vi "電梯2.vi"() -> ()   [LabVIEW 2021]
panel:
  out "時間":string
  out "日期":string
  out "訊息":string
  out "現在樓層":i32
  in  "四樓":bool
  in  "三樓":bool
  in  "二樓":bool
  in  "一樓":bool
  in  "緊急停止":bool
  in  "延長開關":bool
  out "傳感器":bool
  out "樓層位置":i32[](array[numeric])
  in  "程式結束":bool
  out "呼叫樓層":i32
  out "顯示樓層":i32(knob) scale=1.0..4.0
  out "緊急停止燈":bool
  out "顯示燈 4":bool
  out "顯示燈 3":bool
  out "顯示燈 2":bool
  out "顯示燈":bool
  out "電梯門 4":u16(ring)
  out "電梯門 3":u16(ring)
  out "電梯門 2":u16(ring)
  out "電梯門":u16(ring)
  out "電梯位置":i32(slide) scale=0.0..4.0
  in  "呼叫鈕4":bool
  in  "呼叫鈕3":bool
  in  "呼叫鈕2":bool
  in  "呼叫鈕":bool
  # "4"
  # "3"
  # "2"
  # "1"
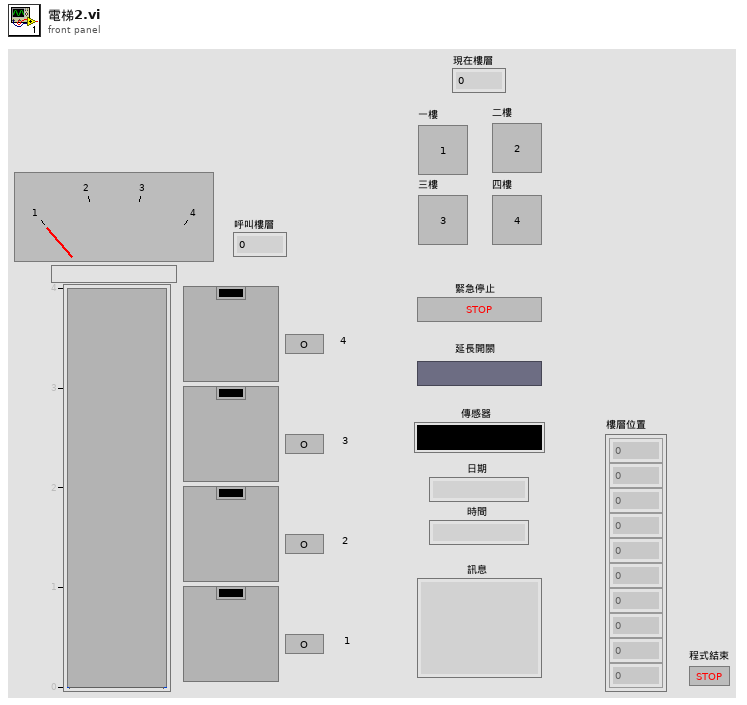
[diagram p1: front panel]
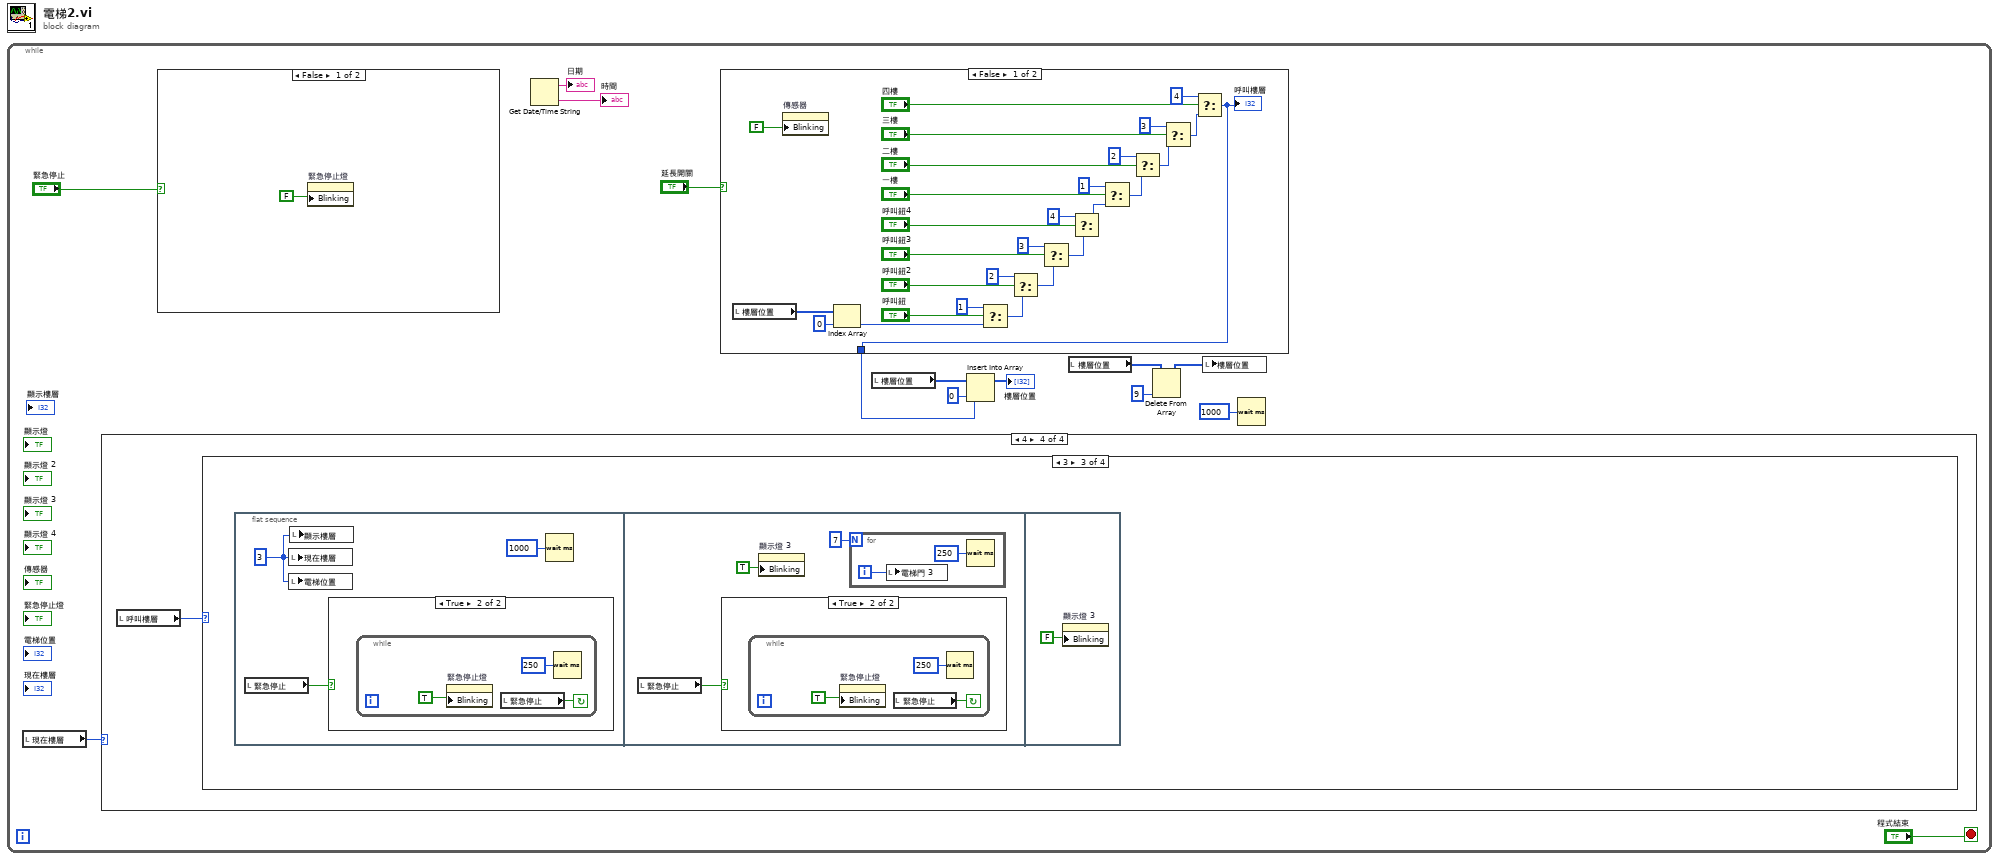
[diagram p0: block diagram]
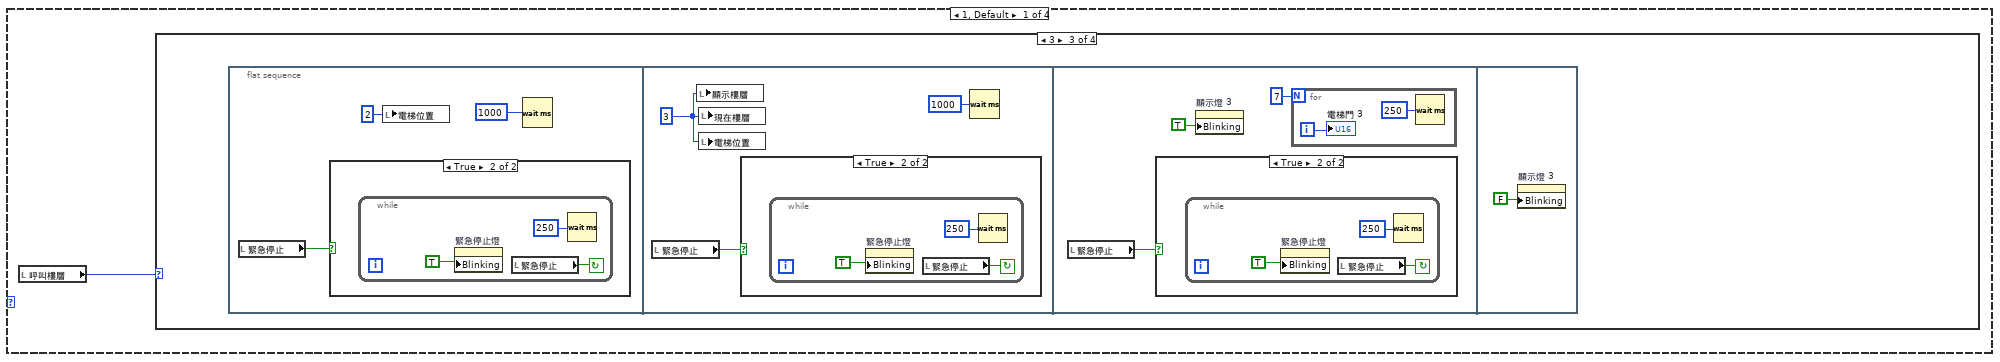
[diagram p2: hidden frame]
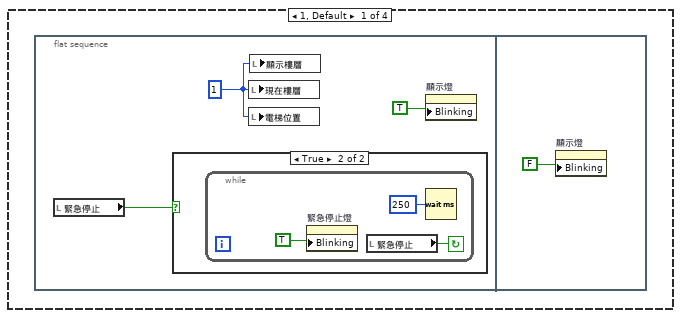
[diagram p3: hidden frame]
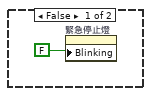
[diagram p4: hidden frame]
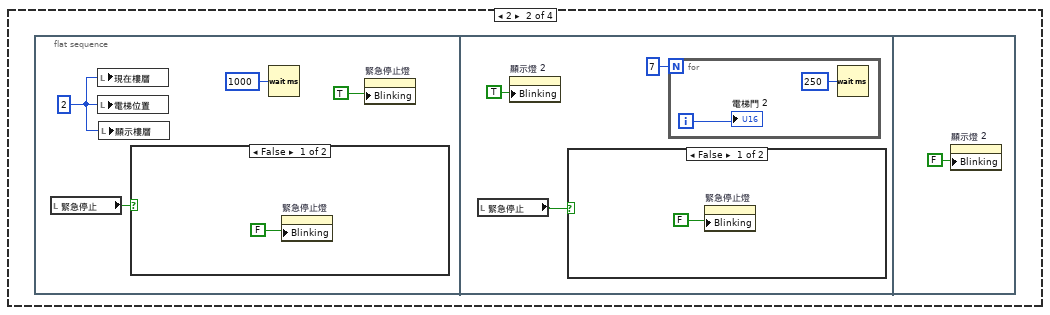
[diagram p5: hidden frame]
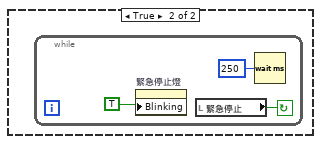
[diagram p6: hidden frame]
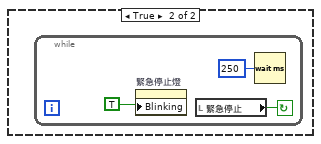
[diagram p7: hidden frame]
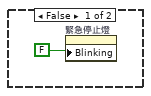
[diagram p8: hidden frame]
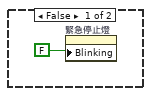
[diagram p9: hidden frame]
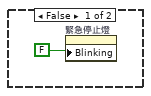
[diagram p10: hidden frame]
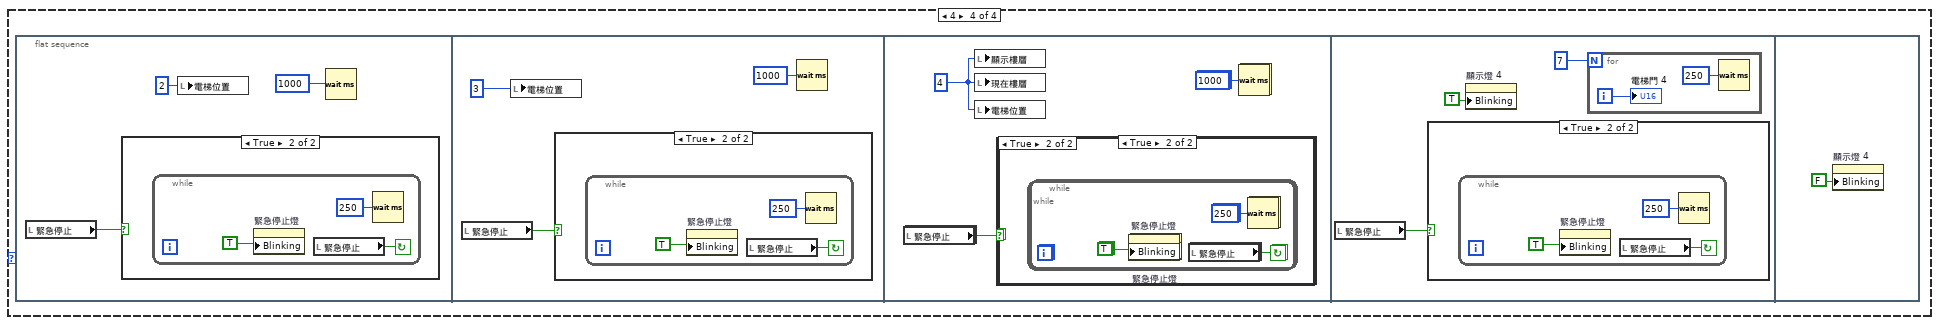
[diagram p11: hidden frame]
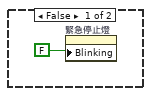
[diagram p12: hidden frame]
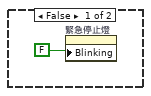
[diagram p13: hidden frame]
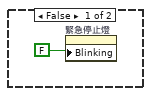
[diagram p14: hidden frame]
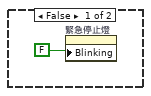
[diagram p15: hidden frame]
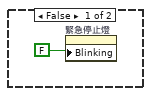
[diagram p16: hidden frame]
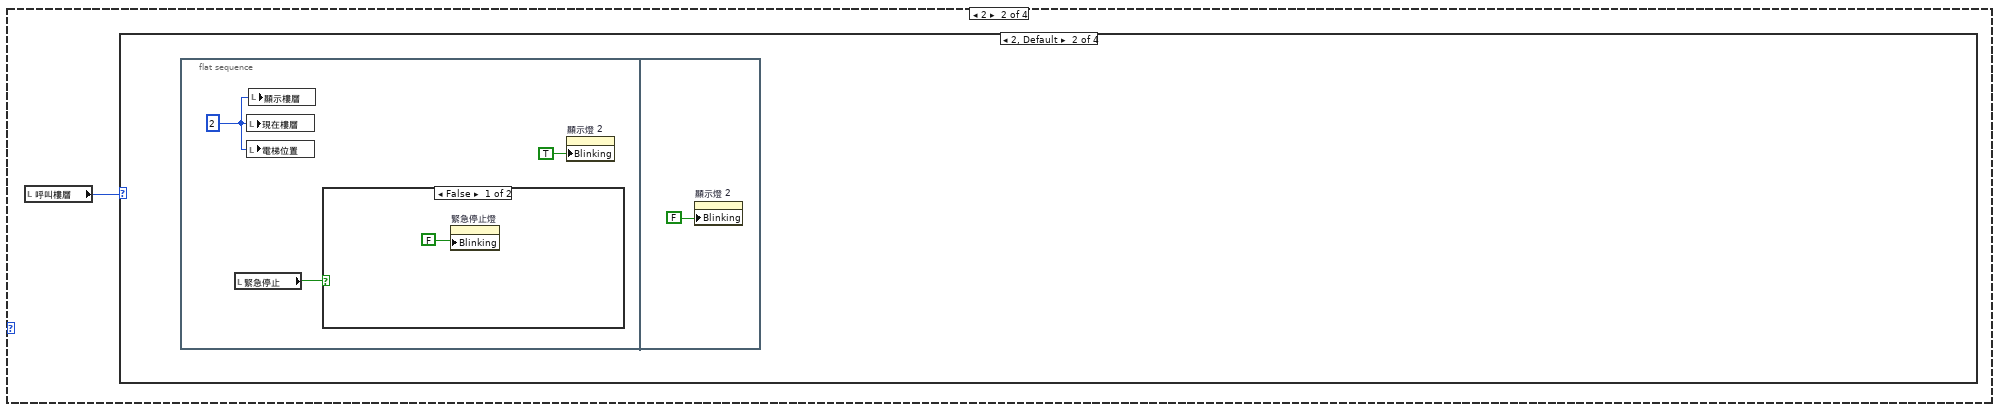
[diagram p17: hidden frame]
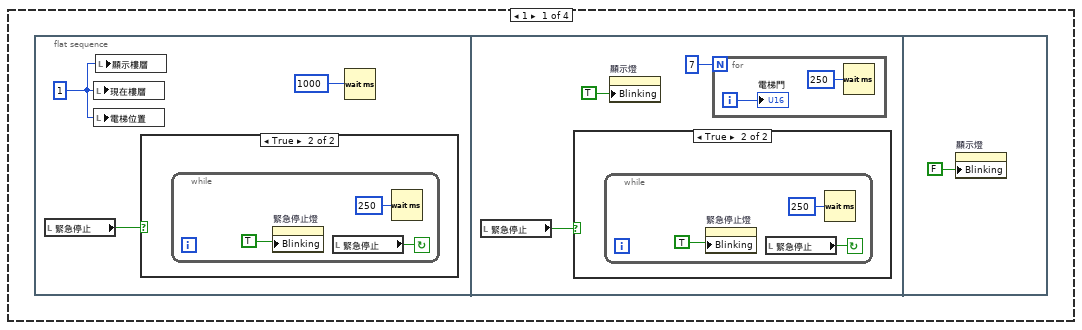
[diagram p18: hidden frame]
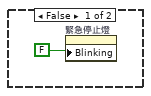
[diagram p19: hidden frame]
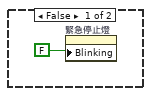
[diagram p20: hidden frame]
diagram:
  n1 = while {
    stop <- "程式結束" stop-if-true
    n2 = local read "現在樓層"() -> (w4:i32)
    n3 = case shown="4" w4 {
      frame 1, Default {
        n4 = local read "呼叫樓層"() -> (w15:i32)
        n5 = case shown="3" w15 {
          frame 1, Default {
            n6 = flat-sequence {
              frame #0 {
                w16 = 1
                n7 = local read "緊急停止"() -> (w18:bool)
                n8 = case shown="True" w18 {
                  frame False {
                    n9 = property on="緊急停止燈" class="Bool (strict)"("Blinking"=FALSE) -> ()  [unwired: 2 in, 2 out]
                  }
                  frame True {
                    n10 = while {
                      stop <- w22 continue-if-true
                      n11 = property on="緊急停止燈" class="Bool (strict)"("Blinking"=TRUE) -> ()  [unwired: 2 in, 2 out]
                      n12 = local read "緊急停止"() -> (w22:bool)
                      n13 = Wait (ms)(milliseconds to wait=u32 250) -> ()  [unwired: 1 out]
                    }
                  }
                }
                n14 = local write "現在樓層"(w16) -> ()
                n15 = local write "電梯位置"(w16) -> ()
                n16 = local write "顯示樓層"(w16) -> ()
                n17 = property on="顯示燈" class="Bool (strict)"("Blinking"=TRUE) -> ()  [unwired: 2 in, 2 out]
              }
              frame #1 {
                n18 = property on="顯示燈" class="Bool (strict)"("Blinking"=FALSE) -> ()  [unwired: 2 in, 2 out]
              }
            }
          }
          frame 2 {
            n19 = flat-sequence {
              frame #0 {
                w24 = 2
                n20 = local read "緊急停止"() -> (w27:bool)
                n21 = local write "現在樓層"(w24) -> ()
                n22 = local write "電梯位置"(w24) -> ()
                n23 = local write "顯示樓層"(w24) -> ()
                n24 = case shown="False" w27 {
                  frame False {
                    n25 = property on="緊急停止燈" class="Bool (strict)"("Blinking"=FALSE) -> ()  [unwired: 2 in, 2 out]
                  }
                  frame True {
                    n26 = while {
                      stop <- w31 continue-if-true
                      n27 = property on="緊急停止燈" class="Bool (strict)"("Blinking"=TRUE) -> ()  [unwired: 2 in, 2 out]
                      n28 = local read "緊急停止"() -> (w31:bool)
                      n29 = Wait (ms)(milliseconds to wait=u32 250) -> ()  [unwired: 1 out]
                    }
                  }
                }
                n30 = Wait (ms)(milliseconds to wait=u32 1000) -> ()  [unwired: 1 out]
                n31 = property on="緊急停止燈" class="Bool (strict)"("Blinking"=TRUE) -> ()  [unwired: 2 in, 2 out]
              }
              frame #1 {
                n32 = local read "緊急停止"() -> (w34:bool)
                n33 = property on="顯示燈 2" class="Bool (strict)"("Blinking"=TRUE) -> ()  [unwired: 2 in, 2 out]
                n34 = case shown="False" w34 {
                  frame False {
                    n35 = property on="緊急停止燈" class="Bool (strict)"("Blinking"=FALSE) -> ()  [unwired: 2 in, 2 out]
                  }
                  frame True {
                    n36 = while {
                      stop <- w40 continue-if-true
                      n37 = property on="緊急停止燈" class="Bool (strict)"("Blinking"=TRUE) -> ()  [unwired: 2 in, 2 out]
                      n38 = local read "緊急停止"() -> (w40:bool)
                      n39 = Wait (ms)(milliseconds to wait=u32 250) -> ()  [unwired: 1 out]
                    }
                  }
                }
                n40 = for {
                  N: 7 -> [_]
                  i -> [w35]
                  n41 = Wait (ms)(milliseconds to wait=u32 250) -> ()  [unwired: 1 out]
                  "電梯門 2" <- w35
                }
              }
              frame #2 {
                n42 = property on="顯示燈 2" class="Bool (strict)"("Blinking"=FALSE) -> ()  [unwired: 2 in, 2 out]
              }
            }
          }
          frame 3 {
            n43 = flat-sequence {
              frame #0 {
                n44 = local read "緊急停止"() -> (w44:bool)
                n45 = case shown="True" w44 {
                  frame False {
                    n46 = property on="緊急停止燈" class="Bool (strict)"("Blinking"=FALSE) -> ()  [unwired: 2 in, 2 out]
                  }
                  frame True {
                    n47 = while {
                      stop <- w48 continue-if-true
                      n48 = property on="緊急停止燈" class="Bool (strict)"("Blinking"=TRUE) -> ()  [unwired: 2 in, 2 out]
                      n49 = local read "緊急停止"() -> (w48:bool)
                      n50 = Wait (ms)(milliseconds to wait=u32 250) -> ()  [unwired: 1 out]
                    }
                  }
                }
                n51 = local write "電梯位置"(2 ("電梯位置")) -> ()
                n52 = Wait (ms)(milliseconds to wait=u32 1000) -> ()  [unwired: 1 out]
              }
              frame #1 {
                w49 = 3
                n53 = local read "緊急停止"() -> (w51:bool)
                n54 = local write "顯示樓層"(w49) -> ()
                n55 = local write "現在樓層"(w49) -> ()
                n56 = local write "電梯位置"(w49) -> ()
                n57 = case shown="True" w51 {
                  frame False {
                    n58 = property on="緊急停止燈" class="Bool (strict)"("Blinking"=FALSE) -> ()  [unwired: 2 in, 2 out]
                  }
                  frame True {
                    n59 = while {
                      stop <- w55 continue-if-true
                      n60 = property on="緊急停止燈" class="Bool (strict)"("Blinking"=TRUE) -> ()  [unwired: 2 in, 2 out]
                      n61 = local read "緊急停止"() -> (w55:bool)
                      n62 = Wait (ms)(milliseconds to wait=u32 250) -> ()  [unwired: 1 out]
                    }
                  }
                }
                n63 = Wait (ms)(milliseconds to wait=u32 1000) -> ()  [unwired: 1 out]
              }
              frame #2 {
                n64 = local read "緊急停止"() -> (w58:bool)
                n65 = case shown="True" w58 {
                  frame False {
                    n66 = property on="緊急停止燈" class="Bool (strict)"("Blinking"=FALSE) -> ()  [unwired: 2 in, 2 out]
                  }
                  frame True {
                    n67 = while {
                      stop <- w64 continue-if-true
                      n68 = property on="緊急停止燈" class="Bool (strict)"("Blinking"=TRUE) -> ()  [unwired: 2 in, 2 out]
                      n69 = local read "緊急停止"() -> (w64:bool)
                      n70 = Wait (ms)(milliseconds to wait=u32 250) -> ()  [unwired: 1 out]
                    }
                  }
                }
                n71 = property on="顯示燈 3" class="Bool (strict)"("Blinking"=TRUE) -> ()  [unwired: 2 in, 2 out]
                n72 = for {
                  N: 7 -> [_]
                  i -> [w60]
                  n73 = Wait (ms)(milliseconds to wait=u32 250) -> ()  [unwired: 1 out]
                  "電梯門 3" <- w60
                }
              }
              frame #3 {
                n74 = property on="顯示燈 3" class="Bool (strict)"("Blinking"=FALSE) -> ()  [unwired: 2 in, 2 out]
              }
            }
          }
          frame 4 {
            n75 = flat-sequence {
              frame #0 {
                n76 = local read "緊急停止"() -> (w68:bool)
                n77 = case shown="True" w68 {
                  frame False {
                    n78 = property on="緊急停止燈" class="Bool (strict)"("Blinking"=FALSE) -> ()  [unwired: 2 in, 2 out]
                  }
                  frame True {
                    n79 = while {
                      stop <- w72 continue-if-true
                      n80 = property on="緊急停止燈" class="Bool (strict)"("Blinking"=TRUE) -> ()  [unwired: 2 in, 2 out]
                      n81 = local read "緊急停止"() -> (w72:bool)
                      n82 = Wait (ms)(milliseconds to wait=u32 250) -> ()  [unwired: 1 out]
                    }
                  }
                }
                n83 = local write "電梯位置"(2 ("電梯位置")) -> ()
                n84 = Wait (ms)(milliseconds to wait=u32 1000) -> ()  [unwired: 1 out]
              }
              frame #1 {
                n85 = local read "緊急停止"() -> (w75:bool)
                n86 = local write "電梯位置"(3) -> ()
                n87 = case shown="True" w75 {
                  frame False {
                    n88 = property on="緊急停止燈" class="Bool (strict)"("Blinking"=FALSE) -> ()  [unwired: 2 in, 2 out]
                  }
                  frame True {
                    n89 = while {
                      stop <- w79 continue-if-true
                      n90 = property on="緊急停止燈" class="Bool (strict)"("Blinking"=TRUE) -> ()  [unwired: 2 in, 2 out]
                      n91 = local read "緊急停止"() -> (w79:bool)
                      n92 = Wait (ms)(milliseconds to wait=u32 250) -> ()  [unwired: 1 out]
                    }
                  }
                }
                n93 = Wait (ms)(milliseconds to wait=u32 1000) -> ()  [unwired: 1 out]
              }
              frame #2 {
                w80 = 4
                n94 = local read "緊急停止"() -> (w83:bool)
                n95 = local read "緊急停止"() -> (w82:bool)
                n96 = local write "顯示樓層"(w80) -> ()
                n97 = local write "現在樓層"(w80) -> ()
                n98 = local write "電梯位置"(w80) -> ()
                n99 = case shown="True" w83 {
                  frame False {
                    n100 = property on="緊急停止燈" class="Bool (strict)"("Blinking"=FALSE) -> ()  [unwired: 2 in, 2 out]
                  }
                  frame True {
                    n101 = while {
                      stop <- w92 continue-if-true
                      n102 = property on="緊急停止燈" class="Bool (strict)"("Blinking"=TRUE) -> ()  [unwired: 2 in, 2 out]
                      n103 = local read "緊急停止"() -> (w92:bool)
                      n104 = Wait (ms)(milliseconds to wait=u32 250) -> ()  [unwired: 1 out]
                    }
                  }
                }
                n105 = case shown="True" w82 {
                  frame False {
                    n106 = property on="緊急停止燈" class="Bool (strict)"("Blinking"=FALSE) -> ()  [unwired: 2 in, 2 out]
                  }
                  frame True {
                    n107 = while {
                      stop <- w88 continue-if-true
                      n108 = property on="緊急停止燈" class="Bool (strict)"("Blinking"=TRUE) -> ()  [unwired: 2 in, 2 out]
                      n109 = local read "緊急停止"() -> (w88:bool)
                      n110 = Wait (ms)(milliseconds to wait=u32 250) -> ()  [unwired: 1 out]
                    }
                  }
                }
                n111 = Wait (ms)(milliseconds to wait=u32 1000) -> ()  [unwired: 1 out]
                n112 = Wait (ms)(milliseconds to wait=u32 1000) -> ()  [unwired: 1 out]
              }
              frame #3 {
                n113 = local read "緊急停止"() -> (w95:bool)
                n114 = case shown="True" w95 {
                  frame False {
                    n115 = property on="緊急停止燈" class="Bool (strict)"("Blinking"=FALSE) -> ()  [unwired: 2 in, 2 out]
                  }
                  frame True {
                    n116 = while {
                      stop <- w101 continue-if-true
                      n117 = property on="緊急停止燈" class="Bool (strict)"("Blinking"=TRUE) -> ()  [unwired: 2 in, 2 out]
                      n118 = local read "緊急停止"() -> (w101:bool)
                      n119 = Wait (ms)(milliseconds to wait=u32 250) -> ()  [unwired: 1 out]
                    }
                  }
                }
                n120 = property on="顯示燈 4" class="Bool (strict)"("Blinking"=TRUE) -> ()  [unwired: 2 in, 2 out]
                n121 = for {
                  N: 7 -> [_]
                  i -> [w96]
                  n122 = Wait (ms)(milliseconds to wait=u32 250) -> ()  [unwired: 1 out]
                  "電梯門 4" <- w96
                }
              }
              frame #4 {
                n123 = property on="顯示燈 4" class="Bool (strict)"("Blinking"=FALSE) -> ()  [unwired: 2 in, 2 out]
              }
            }
          }
        }
      }
      frame 2 {
        n124 = local read "呼叫樓層"() -> (w103:i32)
        n125 = case shown="2, Default" w103 {
          frame 1 {
            n126 = flat-sequence {
              frame #0 {
                w104 = 1
                n127 = local read "緊急停止"() -> (w106:bool)
                n128 = local write "現在樓層"(w104) -> ()
                n129 = local write "電梯位置"(w104) -> ()
                n130 = local write "顯示樓層"(w104) -> ()
                n131 = case shown="True" w106 {
                  frame False {
                    n132 = property on="緊急停止燈" class="Bool (strict)"("Blinking"=FALSE) -> ()  [unwired: 2 in, 2 out]
                  }
                  frame True {
                    n133 = while {
                      stop <- w110 continue-if-true
                      n134 = property on="緊急停止燈" class="Bool (strict)"("Blinking"=TRUE) -> ()  [unwired: 2 in, 2 out]
                      n135 = local read "緊急停止"() -> (w110:bool)
                      n136 = Wait (ms)(milliseconds to wait=u32 250) -> ()  [unwired: 1 out]
                    }
                  }
                }
                n137 = Wait (ms)(milliseconds to wait=u32 1000) -> ()  [unwired: 1 out]
              }
              frame #1 {
                n138 = local read "緊急停止"() -> (w113:bool)
                n139 = case shown="True" w113 {
                  frame False {
                    n140 = property on="緊急停止燈" class="Bool (strict)"("Blinking"=FALSE) -> ()  [unwired: 2 in, 2 out]
                  }
                  frame True {
                    n141 = while {
                      stop <- w119 continue-if-true
                      n142 = property on="緊急停止燈" class="Bool (strict)"("Blinking"=TRUE) -> ()  [unwired: 2 in, 2 out]
                      n143 = local read "緊急停止"() -> (w119:bool)
                      n144 = Wait (ms)(milliseconds to wait=u32 250) -> ()  [unwired: 1 out]
                    }
                  }
                }
                n145 = property on="顯示燈" class="Bool (strict)"("Blinking"=TRUE) -> ()  [unwired: 2 in, 2 out]
                n146 = for {
                  N: 7 -> [_]
                  i -> [w114]
                  n147 = Wait (ms)(milliseconds to wait=u32 250) -> ()  [unwired: 1 out]
                  "電梯門" <- w114
                }
              }
              frame #2 {
                n148 = property on="顯示燈" class="Bool (strict)"("Blinking"=FALSE) -> ()  [unwired: 2 in, 2 out]
              }
            }
          }
          frame 2, Default {
            n149 = flat-sequence {
              frame #0 {
                w121 = 2
                n150 = local read "緊急停止"() -> (w123:bool)
                n151 = local write "現在樓層"(w121) -> ()
                n152 = local write "電梯位置"(w121) -> ()
                n153 = local write "顯示樓層"(w121) -> ()
                n154 = case shown="False" w123 {
                  frame False {
                    n155 = property on="緊急停止燈" class="Bool (strict)"("Blinking"=FALSE) -> ()  [unwired: 2 in, 2 out]
                  }
                  frame True {
                    n156 = while {
                      stop <- w127 continue-if-true
                      n157 = property on="緊急停止燈" class="Bool (strict)"("Blinking"=TRUE) -> ()  [unwired: 2 in, 2 out]
                      n158 = local read "緊急停止"() -> (w127:bool)
                      n159 = Wait (ms)(milliseconds to wait=u32 250) -> ()  [unwired: 1 out]
                    }
                  }
                }
                n160 = property on="顯示燈 2" class="Bool (strict)"("Blinking"=TRUE) -> ()  [unwired: 2 in, 2 out]
              }
              frame #1 {
                n161 = property on="顯示燈 2" class="Bool (strict)"("Blinking"=FALSE) -> ()  [unwired: 2 in, 2 out]
              }
            }
          }
          frame 3 {
            n162 = flat-sequence {
              frame #0 {
                w129 = 3
                n163 = local read "緊急停止"() -> (w130:bool)
                n164 = local write "現在樓層"(w129) -> ()
                n165 = local write "電梯位置"(w129) -> ()
                n166 = local write "顯示樓層"(w129) -> ()
                n167 = case shown="True" w130 {
                  frame False {
                    n168 = property on="緊急停止燈" class="Bool (strict)"("Blinking"=FALSE) -> ()  [unwired: 2 in, 2 out]
                  }
                  frame True {
                    n169 = while {
                      stop <- w135 continue-if-true
                      n170 = property on="緊急停止燈" class="Bool (strict)"("Blinking"=TRUE) -> ()  [unwired: 2 in, 2 out]
                      n171 = local read "緊急停止"() -> (w135:bool)
                      n172 = Wait (ms)(milliseconds to wait=u32 250) -> ()  [unwired: 1 out]
                    }
                  }
                }
                n173 = Wait (ms)(milliseconds to wait=u32 1000) -> ()  [unwired: 1 out]
              }
              frame #1 {
                n174 = local read "緊急停止"() -> (w136:bool)
                n175 = case shown="True" w136 {
                  frame False {
                    n176 = property on="緊急停止燈" class="Bool (strict)"("Blinking"=FALSE) -> ()  [unwired: 2 in, 2 out]
                  }
                  frame True {
                    n177 = while {
                      stop <- w144 continue-if-true
                      n178 = property on="緊急停止燈" class="Bool (strict)"("Blinking"=TRUE) -> ()  [unwired: 2 in, 2 out]
                      n179 = local read "緊急停止"() -> (w144:bool)
                      n180 = Wait (ms)(milliseconds to wait=u32 250) -> ()  [unwired: 1 out]
                    }
                  }
                }
                n181 = property on="顯示燈 3" class="Bool (strict)"("Blinking"=TRUE) -> ()  [unwired: 2 in, 2 out]
                n182 = for {
                  N: 7 -> [_]
                  i -> [w139]
                  n183 = local write "電梯門 3"(w139) -> ()
                  n184 = Wait (ms)(milliseconds to wait=u32 250) -> ()  [unwired: 1 out]
                }
              }
              frame #2 {
                n185 = property on="顯示燈 3" class="Bool (strict)"("Blinking"=FALSE) -> ()  [unwired: 2 in, 2 out]
              }
            }
          }
          frame 4 {
            n186 = flat-sequence {
              frame #0 {
                n187 = local read "緊急停止"() -> (w148:bool)
                n188 = case shown="True" w148 {
                  frame False {
                    n189 = property on="緊急停止燈" class="Bool (strict)"("Blinking"=FALSE) -> ()  [unwired: 2 in, 2 out]
                  }
                  frame True {
                    n190 = while {
                      stop <- w152 continue-if-true
                      n191 = property on="緊急停止燈" class="Bool (strict)"("Blinking"=TRUE) -> ()  [unwired: 2 in, 2 out]
                      n192 = local read "緊急停止"() -> (w152:bool)
                      n193 = Wait (ms)(milliseconds to wait=u32 250) -> ()  [unwired: 1 out]
                    }
                  }
                }
                n194 = local write "電梯位置"(3 ("電梯位置")) -> ()
                n195 = Wait (ms)(milliseconds to wait=u32 1000) -> ()  [unwired: 1 out]
              }
              frame #1 {
                w153 = 4
                n196 = local read "緊急停止"() -> (w155:bool)
                n197 = local write "現在樓層"(w153) -> ()
                n198 = local write "電梯位置"(w153) -> ()
                n199 = local write "顯示樓層"(w153) -> ()
                n200 = case shown="True" w155 {
                  frame False {
                    n201 = property on="緊急停止燈" class="Bool (strict)"("Blinking"=FALSE) -> ()  [unwired: 2 in, 2 out]
                  }
                  frame True {
                    n202 = while {
                      stop <- w159 continue-if-true
                      n203 = property on="緊急停止燈" class="Bool (strict)"("Blinking"=TRUE) -> ()  [unwired: 2 in, 2 out]
                      n204 = local read "緊急停止"() -> (w159:bool)
                      n205 = Wait (ms)(milliseconds to wait=u32 250) -> ()  [unwired: 1 out]
                    }
                  }
                }
                n206 = Wait (ms)(milliseconds to wait=u32 1000) -> ()  [unwired: 1 out]
              }
              frame #2 {
                n207 = local read "緊急停止"() -> (w162:bool)
                n208 = case shown="True" w162 {
                  frame False {
                    n209 = property on="緊急停止燈" class="Bool (strict)"("Blinking"=FALSE) -> ()  [unwired: 2 in, 2 out]
                  }
                  frame True {
                    n210 = while {
                      stop <- w168 continue-if-true
                      n211 = property on="緊急停止燈" class="Bool (strict)"("Blinking"=TRUE) -> ()  [unwired: 2 in, 2 out]
                      n212 = local read "緊急停止"() -> (w168:bool)
                      n213 = Wait (ms)(milliseconds to wait=u32 250) -> ()  [unwired: 1 out]
                    }
                  }
                }
                n214 = property on="顯示燈 4" class="Bool (strict)"("Blinking"=TRUE) -> ()  [unwired: 2 in, 2 out]
                n215 = for {
                  N: 7 -> [_]
                  i -> [w163]
                  n216 = local write "電梯門 4"(w163) -> ()
                  n217 = Wait (ms)(milliseconds to wait=u32 250) -> ()  [unwired: 1 out]
                }
              }
              frame #3 {
                n218 = property on="顯示燈 4" class="Bool (strict)"("Blinking"=FALSE) -> ()  [unwired: 2 in, 2 out]
              }
            }
          }
        }
      }
      frame 3 {
        n219 = local read "呼叫樓層"() -> (w170:i32)
        n220 = case shown="4" w170 {
          frame 1 {
            n221 = flat-sequence {
              frame #0 {
                n222 = local read "緊急停止"() -> (w173:bool)
                n223 = case shown="True" w173 {
                  frame False {
                    n224 = property on="緊急停止燈" class="Bool (strict)"("Blinking"=FALSE) -> ()  [unwired: 2 in, 2 out]
                  }
                  frame True {
                    n225 = while {
                      stop <- w177 continue-if-true
                      n226 = property on="緊急停止燈" class="Bool (strict)"("Blinking"=TRUE) -> ()  [unwired: 2 in, 2 out]
                      n227 = local read "緊急停止"() -> (w177:bool)
                      n228 = Wait (ms)(milliseconds to wait=u32 250) -> ()  [unwired: 1 out]
                    }
                  }
                }
                n229 = local write "電梯位置"(2 ("電梯位置")) -> ()
                n230 = Wait (ms)(milliseconds to wait=u32 1000) -> ()  [unwired: 1 out]
              }
              frame #1 {
                w178 = 1
                n231 = local read "緊急停止"() -> (w180:bool)
                n232 = local write "現在樓層"(w178) -> ()
                n233 = local write "電梯位置"(w178) -> ()
                n234 = local write "顯示樓層"(w178) -> ()
                n235 = case shown="True" w180 {
                  frame False {
                    n236 = property on="緊急停止燈" class="Bool (strict)"("Blinking"=FALSE) -> ()  [unwired: 2 in, 2 out]
                  }
                  frame True {
                    n237 = while {
                      stop <- w184 continue-if-true
                      n238 = property on="緊急停止燈" class="Bool (strict)"("Blinking"=TRUE) -> ()  [unwired: 2 in, 2 out]
                      n239 = local read "緊急停止"() -> (w184:bool)
                      n240 = Wait (ms)(milliseconds to wait=u32 250) -> ()  [unwired: 1 out]
                    }
                  }
                }
                n241 = Wait (ms)(milliseconds to wait=u32 1000) -> ()  [unwired: 1 out]
              }
              frame #2 {
                n242 = local read "緊急停止"() -> (w187:bool)
                n243 = case shown="True" w187 {
                  frame False {
                    n244 = property on="緊急停止燈" class="Bool (strict)"("Blinking"=FALSE) -> ()  [unwired: 2 in, 2 out]
                  }
                  frame True {
                    n245 = while {
                      stop <- w193 continue-if-true
                      n246 = property on="緊急停止燈" class="Bool (strict)"("Blinking"=TRUE) -> ()  [unwired: 2 in, 2 out]
                      n247 = local read "緊急停止"() -> (w193:bool)
                      n248 = Wait (ms)(milliseconds to wait=u32 250) -> ()  [unwired: 1 out]
                    }
                  }
                }
                n249 = property on="顯示燈" class="Bool (strict)"("Blinking"=TRUE) -> ()  [unwired: 2 in, 2 out]
                n250 = for {
                  N: 7 -> [_]
                  i -> [w188]
                  n251 = local write "電梯門"(w188) -> ()
                  n252 = Wait (ms)(milliseconds to wait=u32 250) -> ()  [unwired: 1 out]
                }
              }
              frame #3 {
                n253 = property on="顯示燈" class="Bool (strict)"("Blinking"=FALSE) -> ()  [unwired: 2 in, 2 out]
              }
            }
          }
          frame 2 {
            n254 = flat-sequence {
              frame #0 {
                w195 = 2
                n255 = local read "緊急停止"() -> (w197:bool)
                n256 = local write "現在樓層"(w195) -> ()
                n257 = local write "電梯位置"(w195) -> ()
                n258 = local write "顯示樓層"(w195) -> ()
                n259 = case shown="True" w197 {
                  frame False {
                    n260 = property on="緊急停止燈" class="Bool (strict)"("Blinking"=FALSE) -> ()  [unwired: 2 in, 2 out]
                  }
                  frame True {
                    n261 = while {
                      stop <- w201 continue-if-true
                      n262 = property on="緊急停止燈" class="Bool (strict)"("Blinking"=TRUE) -> ()  [unwired: 2 in, 2 out]
                      n263 = local read "緊急停止"() -> (w201:bool)
                      n264 = Wait (ms)(milliseconds to wait=u32 250) -> ()  [unwired: 1 out]
                    }
                  }
                }
                n265 = Wait (ms)(milliseconds to wait=u32 1000) -> ()  [unwired: 1 out]
              }
              frame #1 {
                n266 = local read "緊急停止"() -> (w204:bool)
                n267 = case shown="True" w204 {
                  frame False {
                    n268 = property on="緊急停止燈" class="Bool (strict)"("Blinking"=FALSE) -> ()  [unwired: 2 in, 2 out]
                  }
                  frame True {
                    n269 = while {
                      stop <- w210 continue-if-true
                      n270 = property on="緊急停止燈" class="Bool (strict)"("Blinking"=TRUE) -> ()  [unwired: 2 in, 2 out]
                      n271 = local read "緊急停止"() -> (w210:bool)
                      n272 = Wait (ms)(milliseconds to wait=u32 250) -> ()  [unwired: 1 out]
                    }
                  }
                }
                n273 = property on="顯示燈 2" class="Bool (strict)"("Blinking"=TRUE) -> ()  [unwired: 2 in, 2 out]
                n274 = for {
                  N: 7 -> [_]
                  i -> [w205]
                  n275 = local write "電梯門 2"(w205) -> ()
                  n276 = Wait (ms)(milliseconds to wait=u32 250) -> ()  [unwired: 1 out]
                }
              }
              frame #2 {
                n277 = property on="顯示燈 2" class="Bool (strict)"("Blinking"=FALSE) -> ()  [unwired: 2 in, 2 out]
              }
            }
          }
          frame 3, Default {
            n278 = flat-sequence {
              frame #0 {
                w212 = 3
                n279 = local read "緊急停止"() -> (w214:bool)
                n280 = local write "現在樓層"(w212) -> ()
                n281 = local write "電梯位置"(w212) -> ()
                n282 = local write "顯示樓層"(w212) -> ()
                n283 = case shown="True" w214 {
                  frame False {
                    n284 = property on="緊急停止燈" class="Bool (strict)"("Blinking"=FALSE) -> ()  [unwired: 2 in, 2 out]
                  }
                  frame True {
                    n285 = while {
                      stop <- w218 continue-if-true
                      n286 = property on="緊急停止燈" class="Bool (strict)"("Blinking"=TRUE) -> ()  [unwired: 2 in, 2 out]
                      n287 = local read "緊急停止"() -> (w218:bool)
                      n288 = Wait (ms)(milliseconds to wait=u32 250) -> ()  [unwired: 1 out]
                    }
                  }
                }
                n289 = property on="顯示燈 3" class="Bool (strict)"("Blinking"=TRUE) -> ()  [unwired: 2 in, 2 out]
              }
              frame #1 {
                n290 = property on="顯示燈 3" class="Bool (strict)"("Blinking"=FALSE) -> ()  [unwired: 2 in, 2 out]
              }
            }
          }
          frame 4 {
            n291 = flat-sequence {
              frame #0 {
                w220 = 4
                n292 = local read "緊急停止"() -> (w222:bool)
                n293 = local write "現在樓層"(w220) -> ()
                n294 = local write "電梯位置"(w220) -> ()
                n295 = local write "顯示樓層"(w220) -> ()
                n296 = case shown="True" w222 {
                  frame False {
                    n297 = property on="緊急停止燈" class="Bool (strict)"("Blinking"=FALSE) -> ()  [unwired: 2 in, 2 out]
                  }
                  frame True {
                    n298 = while {
                      stop <- w226 continue-if-true
                      n299 = property on="緊急停止燈" class="Bool (strict)"("Blinking"=TRUE) -> ()  [unwired: 2 in, 2 out]
                      n300 = local read "緊急停止"() -> (w226:bool)
                      n301 = Wait (ms)(milliseconds to wait=u32 250) -> ()  [unwired: 1 out]
                    }
                  }
                }
                n302 = Wait (ms)(milliseconds to wait=u32 1000) -> ()  [unwired: 1 out]
              }
              frame #1 {
                n303 = local read "緊急停止"() -> (w229:bool)
                n304 = case shown="True" w229 {
                  frame False {
                    n305 = property on="緊急停止燈" class="Bool (strict)"("Blinking"=FALSE) -> ()  [unwired: 2 in, 2 out]
                  }
                  frame True {
                    n306 = while {
                      stop <- w235 continue-if-true
                      n307 = property on="緊急停止燈" class="Bool (strict)"("Blinking"=TRUE) -> ()  [unwired: 2 in, 2 out]
                      n308 = local read "緊急停止"() -> (w235:bool)
                      n309 = Wait (ms)(milliseconds to wait=u32 250) -> ()  [unwired: 1 out]
                    }
                  }
                }
                n310 = property on="顯示燈 4" class="Bool (strict)"("Blinking"=TRUE) -> ()  [unwired: 2 in, 2 out]
                n311 = for {
                  N: 7 -> [_]
                  i -> [w230]
                  n312 = local write "電梯門 4"(w230) -> ()
                  n313 = Wait (ms)(milliseconds to wait=u32 250) -> ()  [unwired: 1 out]
                }
              }
              frame #2 {
                n314 = property on="顯示燈 4" class="Bool (strict)"("Blinking"=FALSE) -> ()  [unwired: 2 in, 2 out]
              }
            }
          }
        }
      }
      frame 4 {
        n315 = local read "呼叫樓層"() -> (w237:i32)
        n316 = case shown="3" w237 {
          frame 1 {
            n317 = flat-sequence {
              frame #0 {
                n318 = local read "緊急停止"() -> (w240:bool)
                n319 = case shown="True" w240 {
                  frame False {
                    n320 = property on="緊急停止燈" class="Bool (strict)"("Blinking"=FALSE) -> ()  [unwired: 2 in, 2 out]
                  }
                  frame True {
                    n321 = while {
                      stop <- w244 continue-if-true
                      n322 = property on="緊急停止燈" class="Bool (strict)"("Blinking"=TRUE) -> ()  [unwired: 2 in, 2 out]
                      n323 = local read "緊急停止"() -> (w244:bool)
                      n324 = Wait (ms)(milliseconds to wait=u32 250) -> ()  [unwired: 1 out]
                    }
                  }
                }
                n325 = local write "電梯位置"(3 ("電梯位置")) -> ()
                n326 = Wait (ms)(milliseconds to wait=u32 1000) -> ()  [unwired: 1 out]
              }
              frame #1 {
                n327 = local read "緊急停止"() -> (w247:bool)
                n328 = local write "電梯位置"(2 ("電梯位置")) -> ()
                n329 = case shown="True" w247 {
                  frame False {
                    n330 = property on="緊急停止燈" class="Bool (strict)"("Blinking"=FALSE) -> ()  [unwired: 2 in, 2 out]
                  }
                  frame True {
                    n331 = while {
                      stop <- w251 continue-if-true
                      n332 = property on="緊急停止燈" class="Bool (strict)"("Blinking"=TRUE) -> ()  [unwired: 2 in, 2 out]
                      n333 = local read "緊急停止"() -> (w251:bool)
                      n334 = Wait (ms)(milliseconds to wait=u32 250) -> ()  [unwired: 1 out]
                    }
                  }
                }
                n335 = Wait (ms)(milliseconds to wait=u32 1000) -> ()  [unwired: 1 out]
              }
              frame #2 {
                w252 = 1
                n336 = local read "緊急停止"() -> (w253:bool)
                n337 = local write "現在樓層"(w252) -> ()
                n338 = local write "電梯位置"(w252) -> ()
                n339 = local write "顯示樓層"(w252) -> ()
                n340 = case shown="True" w253 {
                  frame False {
                    n341 = property on="緊急停止燈" class="Bool (strict)"("Blinking"=FALSE) -> ()  [unwired: 2 in, 2 out]
                  }
                  frame True {
                    n342 = while {
                      stop <- w258 continue-if-true
                      n343 = property on="緊急停止燈" class="Bool (strict)"("Blinking"=TRUE) -> ()  [unwired: 2 in, 2 out]
                      n344 = local read "緊急停止"() -> (w258:bool)
                      n345 = Wait (ms)(milliseconds to wait=u32 250) -> ()  [unwired: 1 out]
                    }
                  }
                }
                n346 = Wait (ms)(milliseconds to wait=u32 1000) -> ()  [unwired: 1 out]
              }
              frame #3 {
                n347 = local read "緊急停止"() -> (w261:bool)
                n348 = case shown="True" w261 {
                  frame False {
                    n349 = property on="緊急停止燈" class="Bool (strict)"("Blinking"=FALSE) -> ()  [unwired: 2 in, 2 out]
                  }
                  frame True {
                    n350 = while {
                      stop <- w267 continue-if-true
                      n351 = property on="緊急停止燈" class="Bool (strict)"("Blinking"=TRUE) -> ()  [unwired: 2 in, 2 out]
                      n352 = local read "緊急停止"() -> (w267:bool)
                      n353 = Wait (ms)(milliseconds to wait=u32 250) -> ()  [unwired: 1 out]
                    }
                  }
                }
                n354 = property on="顯示燈" class="Bool (strict)"("Blinking"=TRUE) -> ()  [unwired: 2 in, 2 out]
                n355 = for {
                  N: 7 -> [_]
                  i -> [w262]
                  n356 = local write "電梯門"(w262) -> ()
                  n357 = Wait (ms)(milliseconds to wait=u32 250) -> ()  [unwired: 1 out]
                }
              }
              frame #4 {
                n358 = property on="顯示燈" class="Bool (strict)"("Blinking"=FALSE) -> ()  [unwired: 2 in, 2 out]
              }
            }
          }
          frame 2 {
            n359 = flat-sequence {
              frame #0 {
                n360 = local read "緊急停止"() -> (w271:bool)
                n361 = case shown="True" w271 {
                  frame False {
                    n362 = property on="緊急停止燈" class="Bool (strict)"("Blinking"=FALSE) -> ()  [unwired: 2 in, 2 out]
                  }
                  frame True {
                    n363 = while {
                      stop <- w275 continue-if-true
                      n364 = property on="緊急停止燈" class="Bool (strict)"("Blinking"=TRUE) -> ()  [unwired: 2 in, 2 out]
                      n365 = local read "緊急停止"() -> (w275:bool)
                      n366 = Wait (ms)(milliseconds to wait=u32 250) -> ()  [unwired: 1 out]
                    }
                  }
                }
                n367 = local write "電梯位置"(3 ("電梯位置")) -> ()
                n368 = Wait (ms)(milliseconds to wait=u32 1000) -> ()  [unwired: 1 out]
              }
              frame #1 {
                w276 = 2
                n369 = local read "緊急停止"() -> (w278:bool)
                n370 = local write "現在樓層"(w276) -> ()
                n371 = local write "電梯位置"(w276) -> ()
                n372 = local write "顯示樓層"(w276) -> ()
                n373 = case shown="True" w278 {
                  frame False {
                    n374 = property on="緊急停止燈" class="Bool (strict)"("Blinking"=FALSE) -> ()  [unwired: 2 in, 2 out]
                  }
                  frame True {
                    n375 = while {
                      stop <- w282 continue-if-true
                      n376 = property on="緊急停止燈" class="Bool (strict)"("Blinking"=TRUE) -> ()  [unwired: 2 in, 2 out]
                      n377 = local read "緊急停止"() -> (w282:bool)
                      n378 = Wait (ms)(milliseconds to wait=u32 250) -> ()  [unwired: 1 out]
                    }
                  }
                }
                n379 = Wait (ms)(milliseconds to wait=u32 1000) -> ()  [unwired: 1 out]
              }
              frame #2 {
                n380 = local read "緊急停止"() -> (w285:bool)
                n381 = case shown="True" w285 {
                  frame False {
                    n382 = property on="緊急停止燈" class="Bool (strict)"("Blinking"=FALSE) -> ()  [unwired: 2 in, 2 out]
                  }
                  frame True {
                    n383 = while {
                      stop <- w291 continue-if-true
                      n384 = property on="緊急停止燈" class="Bool (strict)"("Blinking"=TRUE) -> ()  [unwired: 2 in, 2 out]
                      n385 = local read "緊急停止"() -> (w291:bool)
                      n386 = Wait (ms)(milliseconds to wait=u32 250) -> ()  [unwired: 1 out]
                    }
                  }
                }
                n387 = property on="顯示燈 2" class="Bool (strict)"("Blinking"=TRUE) -> ()  [unwired: 2 in, 2 out]
                n388 = for {
                  N: 7 -> [_]
                  i -> [w286]
                  n389 = local write "電梯門 2"(w286) -> ()
                  n390 = Wait (ms)(milliseconds to wait=u32 250) -> ()  [unwired: 1 out]
                }
              }
              frame #3 {
                n391 = property on="顯示燈 2" class="Bool (strict)"("Blinking"=FALSE) -> ()  [unwired: 2 in, 2 out]
              }
            }
          }
          frame 3 {
            n392 = flat-sequence {
              frame #0 {
                w293 = 3
                n393 = local read "緊急停止"() -> (w295:bool)
                n394 = local write "現在樓層"(w293) -> ()
                n395 = local write "電梯位置"(w293) -> ()
                n396 = local write "顯示樓層"(w293) -> ()
                n397 = case shown="True" w295 {
                  frame False {
                    n398 = property on="緊急停止燈" class="Bool (strict)"("Blinking"=FALSE) -> ()  [unwired: 2 in, 2 out]
                  }
                  frame True {
                    n399 = while {
                      stop <- w299 continue-if-true
                      n400 = property on="緊急停止燈" class="Bool (strict)"("Blinking"=TRUE) -> ()  [unwired: 2 in, 2 out]
                      n401 = local read "緊急停止"() -> (w299:bool)
                      n402 = Wait (ms)(milliseconds to wait=u32 250) -> ()  [unwired: 1 out]
                    }
                  }
                }
                n403 = Wait (ms)(milliseconds to wait=u32 1000) -> ()  [unwired: 1 out]
              }
              frame #1 {
                n404 = local read "緊急停止"() -> (w302:bool)
                n405 = case shown="True" w302 {
                  frame False {
                    n406 = property on="緊急停止燈" class="Bool (strict)"("Blinking"=FALSE) -> ()  [unwired: 2 in, 2 out]
                  }
                  frame True {
                    n407 = while {
                      stop <- w308 continue-if-true
                      n408 = property on="緊急停止燈" class="Bool (strict)"("Blinking"=TRUE) -> ()  [unwired: 2 in, 2 out]
                      n409 = local read "緊急停止"() -> (w308:bool)
                      n410 = Wait (ms)(milliseconds to wait=u32 250) -> ()  [unwired: 1 out]
                    }
                  }
                }
                n411 = property on="顯示燈 3" class="Bool (strict)"("Blinking"=TRUE) -> ()  [unwired: 2 in, 2 out]
                n412 = for {
                  N: 7 -> [_]
                  i -> [w303]
                  n413 = local write "電梯門 3"(w303) -> ()
                  n414 = Wait (ms)(milliseconds to wait=u32 250) -> ()  [unwired: 1 out]
                }
              }
              frame #2 {
                n415 = property on="顯示燈 3" class="Bool (strict)"("Blinking"=FALSE) -> ()  [unwired: 2 in, 2 out]
              }
            }
          }
          frame 4, Default {
            n416 = flat-sequence {
              frame #0 {
                w310 = 4
                n417 = local read "緊急停止"() -> (w312:bool)
                n418 = local write "顯示樓層"(w310) -> ()
                n419 = local write "現在樓層"(w310) -> ()
                n420 = local write "電梯位置"(w310) -> ()
                n421 = case shown="True" w312 {
                  frame False {
                    n422 = property on="緊急停止燈" class="Bool (strict)"("Blinking"=FALSE) -> ()  [unwired: 2 in, 2 out]
                  }
                  frame True {
                    n423 = while {
                      stop <- w316 continue-if-true
                      n424 = property on="緊急停止燈" class="Bool (strict)"("Blinking"=TRUE) -> ()  [unwired: 2 in, 2 out]
                      n425 = local read "緊急停止"() -> (w316:bool)
                      n426 = Wait (ms)(milliseconds to wait=u32 250) -> ()  [unwired: 1 out]
                    }
                  }
                }
                n427 = property on="顯示燈 4" class="Bool (strict)"("Blinking"=TRUE) -> ()  [unwired: 2 in, 2 out]
              }
              frame #1 {
                n428 = property on="顯示燈 4" class="Bool (strict)"("Blinking"=FALSE) -> ()  [unwired: 2 in, 2 out]
              }
            }
          }
        }
      }
    }
    n429 = case shown="False" "緊急停止" {
      frame False {
        n430 = property on="緊急停止燈" class="Bool (strict)"("Blinking"=FALSE) -> ()  [unwired: 2 in, 2 out]
      }
      frame True {
        n431 = local read "現在樓層"() -> (w353:i32)
        n432 = local read "電梯位置"() -> (w352:i32)
        n433 = while {
          shift-right: [w354] -> _
          shift-left: w353 -> [w354]
          shift-right: [w356] -> _
          shift-left: w352 -> [w356]
          stop <- w357 stop-if-true
          n434 = local write "現在樓層"(w354) -> ()
          n435 = local write "電梯位置"(w356) -> ()
          n436 = local write "顯示樓層"(w354) -> ()
          n437 = local read "緊急停止"() -> (w357:bool)
          n438 = Wait (ms)(milliseconds to wait=u32 250) -> ()  [unwired: 1 out]
        }
        n439 = property on="緊急停止燈" class="Bool (strict)"("Blinking"=TRUE) -> ()  [unwired: 2 in, 2 out]
      }
    }
    n440 = Get Date/Time String() -> (date string=→"日期":string, time string=→"時間":string)  [unwired: 3 in]
    n441 = case shown="False" "延長開關" {
      tunnel: [w322 w347] -> w12
      frame False {
        n442 = local read "樓層位置"() -> (w345:i32[])
        n443 = property on="傳感器" class="Bool (strict)"("Blinking"=FALSE) -> ()  [unwired: 2 in, 2 out]
        n444 = Index Array(array=w345, index=0) -> (element=w321:i32)
        n445 = Select(t=1, s="呼叫鈕", f=w321) -> (s? t:f=w333:i32)
        n446 = Select(t=2, s="呼叫鈕2", f=w333) -> (s? t:f=w332:i32)
        n447 = Select(t=3, s="呼叫鈕3", f=w332) -> (s? t:f=w331:i32)
        n448 = Select(t=4, s="呼叫鈕4", f=w331) -> (s? t:f=w334:i32)
        n449 = Select(t=1, s="一樓", f=w334) -> (s? t:f=w335:i32)
        n450 = Select(t=2, s="二樓", f=w335) -> (s? t:f=w336:i32)
        n451 = Select(t=3, s="三樓", f=w336) -> (s? t:f=w337:i32)
        n452 = Select(t=4, s="四樓", f=w337) -> (s? t:f=w322:i32)
        "呼叫樓層" <- w322
      }
      frame True {
        n453 = property on="傳感器" class="Bool (strict)"("Blinking"=TRUE) -> ()  [unwired: 2 in, 2 out]
        n454 = local read "電梯位置"() -> (w347:i32)
        n455 = local write "電梯位置"(w347) -> ()
        n456 = local write "呼叫樓層"(w347) -> ()
        n457 = Wait (ms)(milliseconds to wait=u32 1000) -> ()  [unwired: 1 out]
        "訊息" <- "延長已經開啟，如要運作請將延長開關關閉。" ("message")
      }
    }
    n458 = local read "樓層位置"() -> (w11:i32[])
    n459 = Insert Into Array(array=w11, index=0, new element=w12) -> (→"樓層位置":i32[])
    n460 = local read "樓層位置"() -> (w7:i32[])
    n461 = Delete From Array(array=w7, index=9) -> (array with subset deleted=w5:i32[])  [unwired: 1 in, 1 out]
    n462 = local write "樓層位置"(w5) -> ()
    n463 = Wait (ms)(milliseconds to wait=u32 1000) -> ()  [unwired: 1 out]
  }
